vi "WPI_RobotDriveMecanumMotors.vi"(6 "Rear Right":dbl, 7 "Rear Left":dbl, 8 "error in":errorcluster, 9 "Front Right":dbl, 10 "Front Left":dbl, 11 "RobotDriveDevRef in":T1) -> (0 "error out":errorcluster, 2 "Motor Values":dbl[](array[numeric]), 3 "RobotDriveDevRef out":T1)   [LabVIEW 2017]
doc: "Update each motor with the appropriate power for that wheel."
uses:
  <vilib>/Rock Robotics/WPI/RobotDrive/WPI_RobotDriveDevRef.ctl
  <vilib>/Rock Robotics/WPI/MotorControl/WPI_MotorControlDeviceRef.ctl
  <vilib>/Rock Robotics/WPI/MotorControl/WPI_MotorControlType.ctl
  <vilib>/Rock Robotics/SystemInterfaces/DIO/FPGA_DIOPWMChannel.ctl
  <vilib>/Rock Robotics/WPI/PWM/WPI_PWMDeadband.ctl
  <vilib>/Rock Robotics/SystemInterfaces/DIO/FPGA_DIOChannel.ctl
  <vilib>/Rock Robotics/WPI/RobotDrive/WPI_RobotDriveSafetyCheck.vi
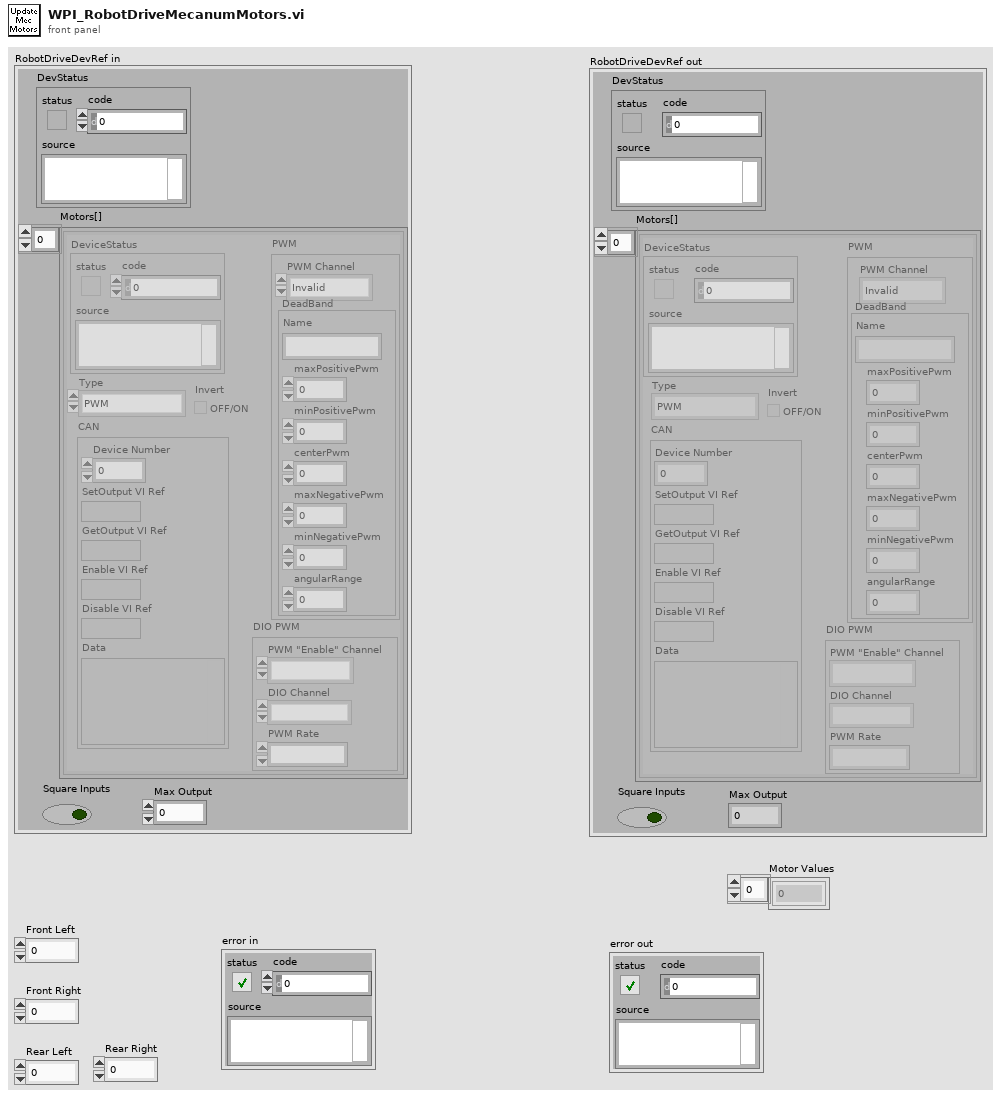
[diagram p1: front panel]
types:
  T1 = typedef "WPI_RobotDriveDevRef.ctl" = cluster{"DevStatus":errorcluster, "Motors[]":T2[], "Square Inputs":bool, "Max Output":dbl}
  T2 = typedef "WPI_MotorControlDeviceRef.ctl" = cluster{"DeviceStatus":errorcluster, "Type":T3, "PWM":cluster{"PWM Channel":T4, "DeadBand":T5}, "CAN":cluster{"Device Number":u8, "SetOutput VI Ref":variant, "GetOutput VI Ref":variant, "Enable VI Ref":variant, "Disable VI Ref":variant, "Data":variant}, "Invert":bool, "DIO PWM":cluster{"PWM \"Enable\" Channel":T4, "DIOChannel":T6, "PWM Rate":dbl}}
  T3 = typedef "WPI_MotorControlType.ctl" = enum16{"PWM", "CAN", "DIO PWM"}
  T4 = typedef "FPGA_DIOPWMChannel.ctl" = enum8{"PWM 0", "PWM 1", "PWM 2", "PWM 3", "PWM 4", "PWM 5", "PWM 6", "PWM 7", "PWM 8", "PWM 9", "PWM MXP 0", "PWM MXP 1", "PWM MXP 2", "PWM MXP 3", "PWM MXP 4", "PWM MXP 5", "PWM MXP 6", "PWM MXP 7", "PWM MXP 8", "PWM MXP 9", "Invalid"}
  T5 = typedef "WPI_PWMDeadband.ctl" = cluster{"Name":string, "maxPositivePwm":i32, "minPositivePwm":i32, "centerPwm":i32, "maxNegativePwm":i32, "minNegativePwm":i32, "angularRange":u16}
  T6 = typedef "FPGA_DIOChannel.ctl" = enum8{"DIO 0", "DIO 1", "DIO 2", "DIO 3", "DIO 4", "DIO 5", "DIO 6", "DIO 7", "DIO 8", "DIO 9", "DIO MXP 0", "DIO MXP 1", "DIO MXP 2", "DIO MXP 3", "DIO MXP 4", "DIO MXP 5", "DIO MXP 6", "DIO MXP 7", "DIO MXP 8", "DIO MXP 9", "DIO MXP 10", "DIO MXP 11", "DIO MXP 12", "DIO MXP 13", "DIO MXP 14", "DIO MXP 15", "SPI Port CS1", "SPI Port CS2", "SPI Port CS3", "SPI Port MISO", "SPI Port MOSI", "Invalid"}
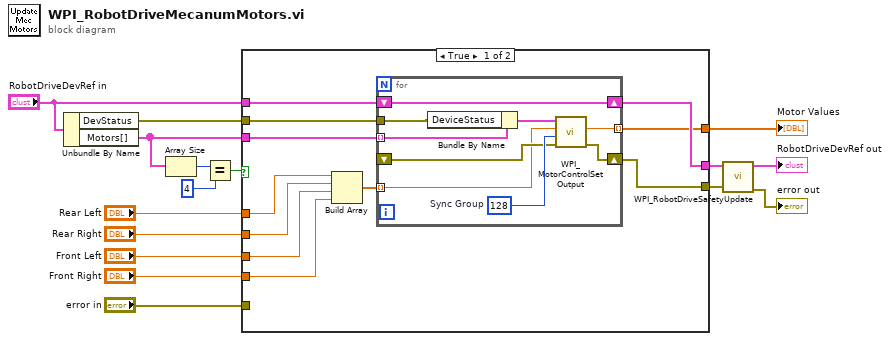
[diagram p0: block diagram]
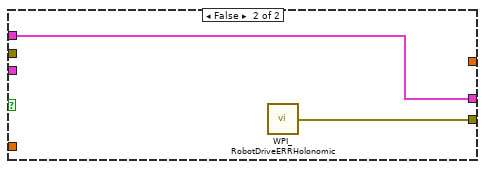
[diagram p2: hidden frame]
diagram:
  n1 = Unbundle By Name("RobotDriveDevRef in") -> ("DevStatus"=w1:errorcluster, "Motors[]"=w2:T2[])
  n2 = Array Size(array=w2) -> (size(s)=w10:i32)
  n3 = Equal?(x=w10, y=4) -> (x = y?=w12:bool)
  n4 = case shown="True" w12 {
    tunnel: "Front Left" -> [w24 _]
    tunnel: "Front Right" -> [w23 _]
    tunnel: [w20 w38] -> w13
    tunnel: "Rear Left" -> [w26 _]
    tunnel: "Rear Right" -> [w25 _]
    tunnel: [w19 _] -> w14
    tunnel: "error in" -> [_ _]
    tunnel: [w21 w37] -> w4
    tunnel: "RobotDriveDevRef in" -> [w22 w37]
    tunnel: w2 -> [w18 _]
    tunnel: w1 -> [w17 _]
    frame True {
      n5 = Build Array(w26, w25, w24, w23) -> (w27:dbl[])
      n6 = for {
        tunnel: [w35] -> w19 mode=indexing
        shift-right: [w34] -> w20
        shift-left: _ -> [w33]
        shift-right: [w32] -> w21
        shift-left: w22 -> [w32]
        tunnel: w18 -> [w29] mode=indexing
        tunnel: w17 -> [w30]
        tunnel: w27 -> [w28] mode=indexing
        w36 = u8 128  # Sync Group
        n7 = Bundle By Name(cluster=w29, "DeviceStatus"=w30) -> (w31:T2)
        n8 = call <vilib>:"WPI_MotorControlSetOutput.vi"("error in (no error)"=w33, "options"=w36, "Output"=w28, "MotorControlDevRef"=w31) -> ("error out"=w34:errorcluster, "Motor Output"=w35:dbl)  [unwired: 1 in, 5 out]
      }
    }
    frame False {
      n9 = call <vilib>:"WPI_RobotDriveERRHolonomic.vi"() -> ("error out"=w38:errorcluster)
    }
  }
  "Motor Values" <- w14
  n10 = call <vilib>:"WPI_RobotDriveSafetyUpdate.vi"("error in (no error)"=w13, "RobotDriveDevRef"=w4) -> ("error out"=→"error out":errorcluster, "RobotDriveDevRef"=→"RobotDriveDevRef out":T1)  [unwired: 8 out]
